vi "cleanup.vi"(4 "error in":errorcluster, 6 "Python session":refnum<k35>) -> (0 "error out":errorcluster)   [LabVIEW 2018]
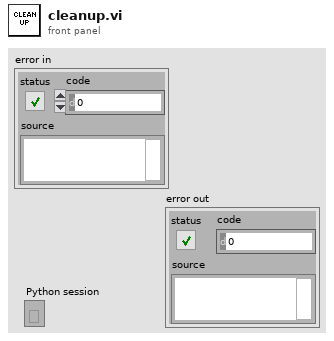
[diagram p1: front panel]
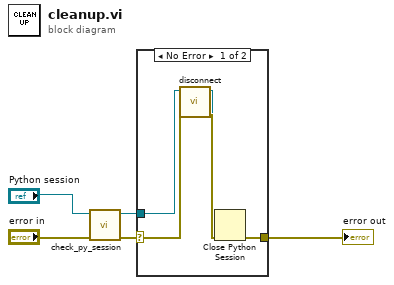
[diagram p0: block diagram]
diagram:
  n1 = call "check_py_session.vi"("error in"="error in", "Python session in"="Python session") -> ("error out"=w3:errorcluster, "Python session out"=w1:refnum<k35>)  [unwired: 3 in, 1 out]
  n2 = case shown="No Error" w3 {
    selector: w3 -> [w8 w11]
    tunnel: [w10 w11] -> w5
    tunnel: w1 -> [w9 _]
    frame No Error {
      n3 = call "disconnect.vi"("error in (no error)"=w8, "Python session in"=w9) -> ("error out"=w7:errorcluster, "Python session out"=w6:refnum<k35>)  [unwired: 3 in, 1 out]
      n4 = Close Python Session(session in=w6, error in=w7) -> (11:w10:errorcluster)
    }
    frame Error {
    }
  }
  "error out" <- w5
